vi "CalcMinPodControlRuntime.vi"(0 "Turret Motor Characteristics":T2={"Free Current"=1.0, "Stall Current"=15.0, "Stall Torque"=10.0, "Free Speed"=10.0, "Gear Ratio"=115.0, "Efficiency"=0.225, "Moment"=2.0}, 1 "Turret Angle Change":dbl=1.0, 2 "Wheel width (m)":dbl=0.01, 3 "Wheel Off-center dist (m)":dbl=0.01, 4 "Max Turret Motor Volts":dbl=10.0, 5 "Drive Magnitude Change":dbl=-5.0, 6 "Drive Motor Characteristics":T2={"Free Current"=1.0, "Stall Current"=15.0, "Stall Torque"=10.0, "Free Speed"=10.0, "Gear Ratio"=115.0, "Efficiency"=0.225, "Moment"=2.0}, 7 "Mass Subset (N)":dbl=60.0, 8 "Pod State Data":T1, 9 "Wheel radius":dbl, 11 "Runtime":dbl) -> (14 "Min. Runtime":dbl, 15 "Drive Motor Data":T3, 16 "Turret Motor Data":T3)   [LabVIEW 2014]
uses:
  Math/Physics Calculations/SolveMotor_Speed,Torque.vi
panel:
  in  "Turret Loss Torque":dbl
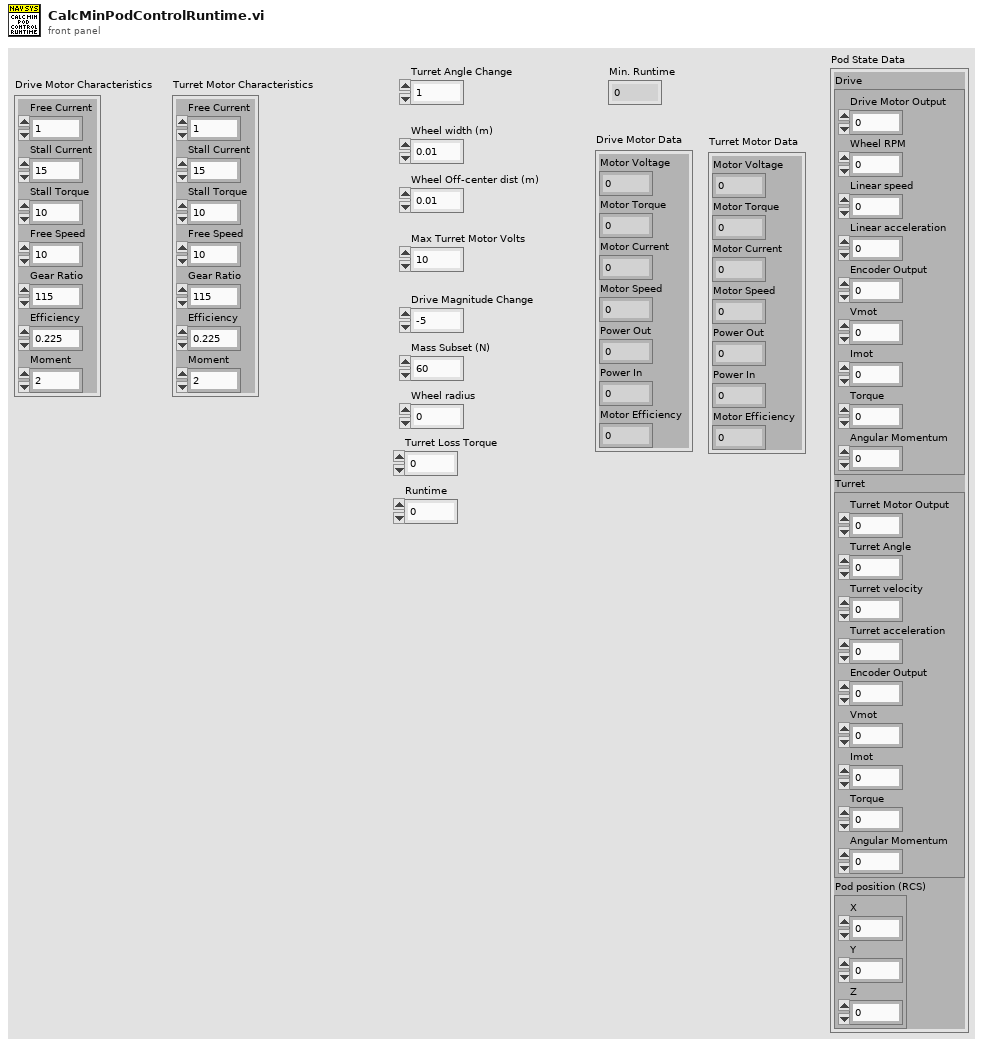
[diagram p1: front panel]
types:
  T1 = cluster{"Drive":cluster{"Drive Motor Output":dbl, "Wheel RPM":dbl, "Linear speed":dbl, "Linear acceleration":dbl, "Encoder Output":dbl, "Vmot":dbl, "Imot":dbl, "Torque":dbl, "Angular Momentum":dbl}, "Turret":cluster{"Turret Motor Output":dbl, "Turret Angle":dbl, "Turret velocity":dbl, "Turret acceleration":dbl, "Encoder Output":dbl, "Vmot":dbl, "Imot":dbl, "Torque":dbl, "Angular Momentum":dbl}, "Pod position (RCS)":cluster{"X":dbl, "Y":dbl, "Z":dbl}}
  T2 = cluster{"Free Current":dbl, "Stall Current":dbl, "Stall Torque":dbl, "Free Speed":dbl, "Gear Ratio":dbl, "Efficiency":dbl, "Moment":dbl}
  T3 = cluster{"Motor Voltage":dbl, "Motor Torque":dbl, "Motor Current":dbl, "Motor Speed":dbl, "Power Out":dbl, "Power In":dbl, "Motor Efficiency":dbl}
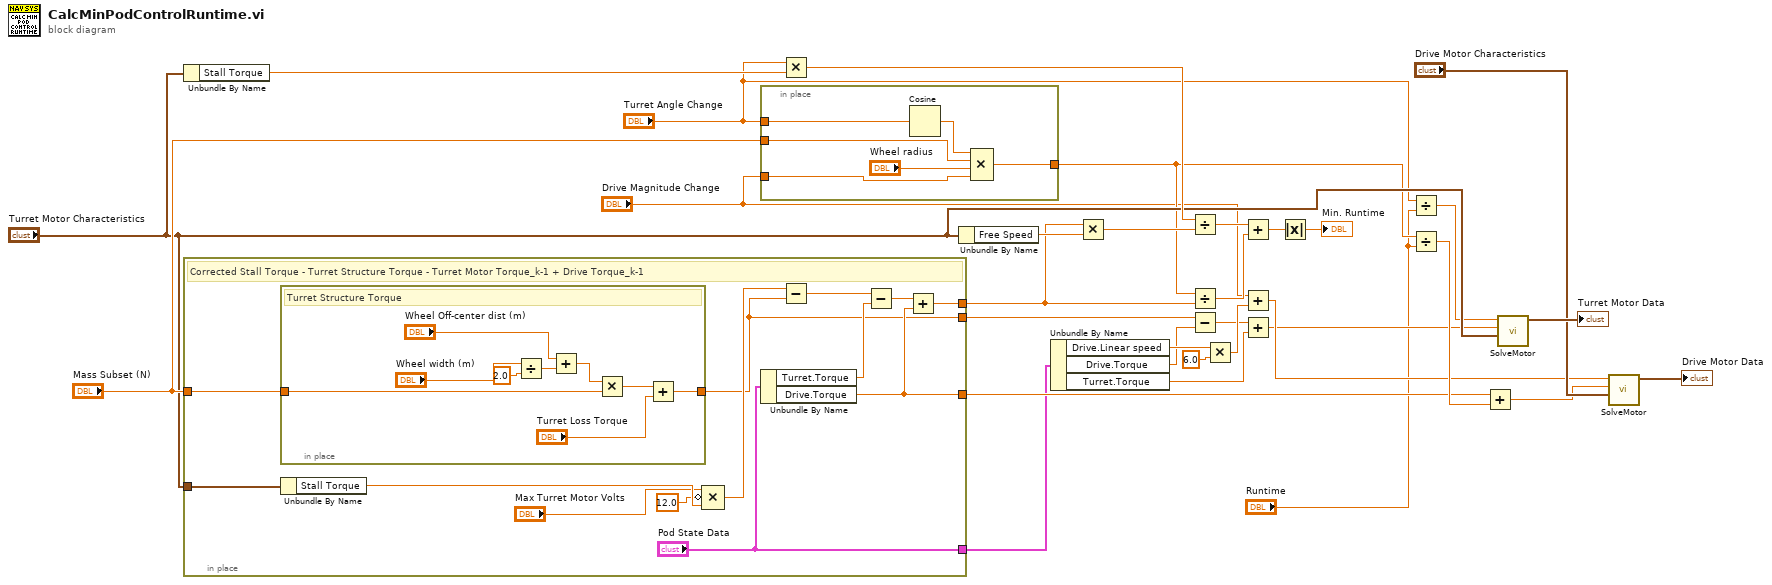
[diagram p0: block diagram]
diagram:
  n1 = Unbundle By Name("Turret Motor Characteristics") -> ("Stall Torque"=w28:dbl)
  n2 = in-place {
    in-place-border: "Turret Motor Characteristics" -> [w45]
    in-place-border: "Mass Subset (N)" -> [w44]
    in-place-border: [w36] -> w23
    in-place-border: [w35] -> w18
    in-place-border: ["Pod State Data"] -> w16
    in-place-border: [w33] -> w7
    # "Corrected Stall Torque - Turret Structure Torque - Turret Motor Torque_k-1 + Drive Torque_k-1"
    n3 = in-place {
      in-place-border: w44 -> [w49]
      in-place-border: [w46] -> w33
      # "Turret Structure Torque"
      n4 = Divide(x="Wheel width (m)", y=2.0) -> (x/y=w52:dbl)
      n5 = Add(x="Wheel Off-center dist (m)", y=w52) -> (x+y=w50:dbl)
      n6 = Multiply(x=w50, y=w49) -> (x*y=w48:dbl)
      n7 = Add(x=w48, y="Turret Loss Torque") -> (x+y=w46:dbl)
    }
    n8 = Unbundle By Name(w45) -> ("Stall Torque"=w43:dbl)
    n9 = Compound Arithmetic op=MULTIPLY("Max Turret Motor Volts", invert 12.0 ("value"), w43) -> (w40:dbl)
    n10 = Unbundle By Name("Pod State Data") -> ("Turret.Torque"=w38:dbl, "Drive.Torque"=w35:dbl)
    n11 = Subtract(x=w40, y=w33) -> (x-y=w39:dbl)
    n12 = Subtract(x=w39, y=w38) -> (x-y=w37:dbl)
    n13 = Add(x=w37, y=w35) -> (x+y=w36:dbl)
  }
  n14 = in-place {
    in-place-border: "Mass Subset (N)" -> [w59]
    in-place-border: [w57] -> w20
    in-place-border: "Turret Angle Change" -> [w56]
    in-place-border: "Drive Magnitude Change" -> [w55]
    n15 = Cosine(x=w56) -> (cos(x)=w60:dbl)
    n16 = Compound Arithmetic op=MULTIPLY(w60, w59, "Wheel radius", w55) -> (w57:dbl)
  }
  n17 = Multiply(x="Turret Angle Change", y=w28) -> (x*y=w26:dbl)
  n18 = Unbundle By Name("Turret Motor Characteristics") -> ("Free Speed"=w29:dbl)
  n19 = Unbundle By Name(w16) -> ("Drive.Linear speed"=w15:dbl, "Drive.Torque"=w8:dbl, "Turret.Torque"=w5:dbl)
  n20 = Multiply(x=w23, y=w29) -> (x*y=w27:dbl)
  n21 = Divide(x=w26, y=w27) -> (x/y=w25:dbl)
  n22 = Divide(x=w20, y=w23) -> (x/y=w22:dbl)
  n23 = Subtract(x=w7, y=w8) -> (x-y=w6:dbl)
  n24 = Multiply(x=w15, y=6.0) -> (x*y=w12:dbl)
  n25 = Add(x=w25, y=w22) -> (x+y=w3:dbl)
  n26 = Add(x="Drive Magnitude Change", y=w12) -> (x+y=w10:dbl)
  n27 = Add(x=w6, y=w5) -> (x+y=w4:dbl)
  n28 = Absolute Value(x=w3) -> (abs(x)=→"Min. Runtime":dbl)
  n29 = Divide(x="Turret Angle Change", y="Runtime") -> (x/y=w9:dbl)
  n30 = Divide(x=w20, y="Runtime") -> (x/y=w19:dbl)
  n31 = Add(x=w18, y=w19) -> (x+y=w17:dbl)
  n32 = call-poly "SolveMotor.vi"("Motor Characteristics"="Turret Motor Characteristics", "Motor Torque"=w4, "Motor Speed"=w9) -> ("Motor Data"=→"Turret Motor Data":T3)  [unwired: 8 in]
  n33 = call-poly "SolveMotor.vi"("Motor Characteristics"="Drive Motor Characteristics", "Motor Torque"=w17, "Motor Speed"=w10) -> ("Motor Data"=→"Drive Motor Data":T3)  [unwired: 8 in]
